vi "Send command Set Pin.vi"(0 "Arduino in":refnum<class "Arduino.lvclass">, 1 "Puerto":string(combo), 2 "Pin":string(combo), 3 "Valor":string(combo), 5 "error in (no error)":errorcluster, 6 "Marca":string) -> (14 "Arduino out":refnum<class "Arduino.lvclass">, 16 "Command":string, 17 "Expected response":string, 19 "error out":errorcluster)   [LabVIEW 2020, in "Arduino.lvclass"]
uses:
  Arduino.lvclass
  Arduino.lvclass/Arduino.ctl
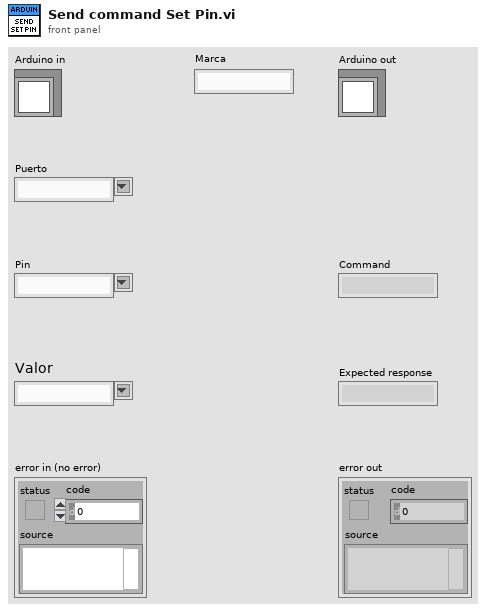
[diagram p1: front panel]
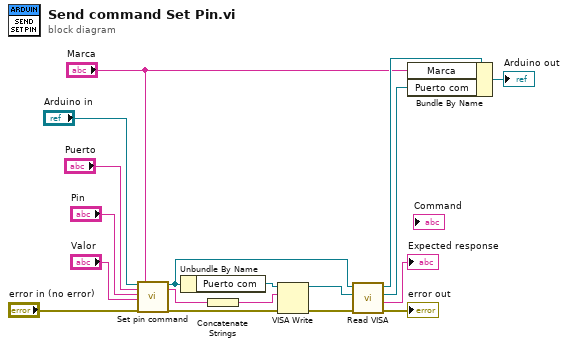
[diagram p0: block diagram]
diagram:
  n1 = call-dynamic "Set pin command.vi"("Serial Device in"="Arduino in", "Puerto"="Puerto", "Pin"="Pin", "Valor"="Valor", "error in (no error)"="error in (no error)", "Marca"="Marca") -> ("Serial Device out"=w8:refnum<class "Arduino.lvclass">, "Command"=w14:string, "error out"=w16:errorcluster)  [unwired: 10 in, 1 out]
  n2 = Unbundle By Name(w8) -> ("Puerto com"=w13:refnum<visa-resource-name>)
  n3 = Concatenate Strings(w14) -> (w15:string)
  n4 = VISA Write(VISA resource name=w13, write buffer=w15, error in (no error)=w16) -> (VISA resource name out=w18:refnum<visa-resource-name>, error out=w17:errorcluster)  [unwired: 1 out]
  n5 = call-dynamic "Read VISA.vi"("error in (no error)"=w17, "VISA Refnum in"=w18, "Serial Device in"=w8) -> ("error out"=→"error out":errorcluster, "Serial Response"=→"Expected response":string, "VISA resource name out"=w9:refnum<visa-resource-name>, "Serial Device out"=w11:refnum<class "Arduino.lvclass">)  [unwired: 5 in]
  n6 = Bundle By Name(cluster=w11, "Marca"="Marca", "Puerto com"=w9) -> (→"Arduino out":refnum<class "Arduino.lvclass">)
